vi "CloseBuild.vi"(8 "error in (no error)":errorcluster, 9 "GeneratedFiles":path[](array[path]), 10 "GeneratedDirectories":path[](array[path]), 11 "Build in":refnum<class "AB_Targetfile.lvclass">) -> (0 "error out":errorcluster, 1 "GeneratedFiles out":path[](array[path]), 3 "Build out":refnum<class "AB_Targetfile.lvclass">)   [LabVIEW 2020, in "AB_Targetfile.lvclass"]
uses:
  <vilib>/AppBuilder/AB_Classes/TargetFile/AB_Targetfile.lvclass
  e:/builds/penguin/labview/branches/2020/dev/dist/vi.lib/AppBuilder/AB_Classes/Build/AB_Build.lvclass
  <vilib>/Utility/error.llb/whitespace.ctl
  <vilib>/AppBuilder/AB_Classes/Build/AB_Build.lvclass
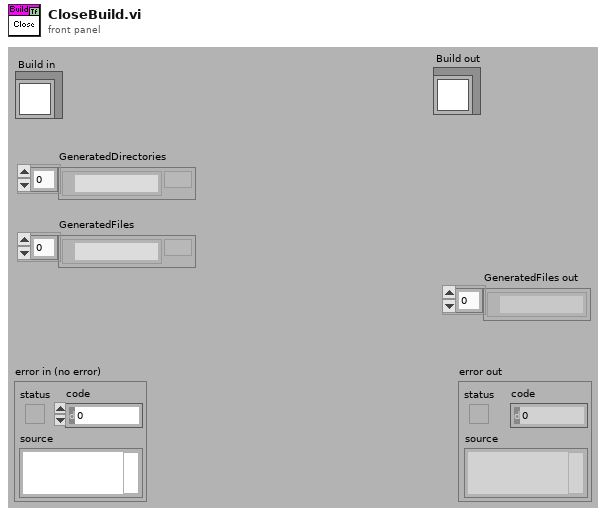
[diagram p1: front panel]
types:
  T1 = typedef "AB_Build.ctl" = cluster{"buildSpecName":string, "buildSpecDescription":string, "destinations":refnum<class "AB_Destination.lvclass">[], "exclusionOption":T2, "defaultLanguage":string, "supportedLanguages":string[], "excludedDirectories":path[], "buildContext":refnum<vi>, "buildObject":T3, "preview":bool, "programatic":bool, "progressBarEvents":T4, "userLog_Path":path, "preActionID":string, "preAction_Path":path, "postActionID":string, "postAction_Path":path, "eng_checkForBrokenVIs?":bool, "eng_verboseLinkerErrors?":bool, "localDest_Path":path, "targetDest_Path":path, "removeVIObject":u16, "cache":refnum<class "PreviewCache.lvclass">, "use cache":bool, "previewCache_ID":string, "buildCache_ID":string, "eng_TempLocalDest_Path":path, "eng_collectDependencies?":bool, "versionInfo":cluster{"buildVersion":cluster{"major":u16, "minor":u16, "patch":u16, "build":u16}, "autoIncrement":bool}, "eng_enableVIChecksums":bool}
  T2 = typedef "AB_Exclusion_Option.ctl" = cluster{"typedefs":bool, "polymorphicVIs":bool, "unusedLibraryItems":bool, "modifyLibraryFile":bool, "edit-timeDependencies":bool, "inlineVIs":bool, "dependent PPLs":bool, "dependent DLLs":bool}
  T3 = typedef "ItemRef.ctl" = u64
  T4 = typedef "provcom_ProgressBar_Events.ctl" = cluster{"newJob":refnum<user-event>, "newItem":refnum<user-event>, "errorMsg":T5, "cancel":refnum<user-event>}
  T5 = typedef "mxLvBuildError.ctl" = refnum<user-event>
  T6 = cluster{"major":u16, "minor":u16, "patch":u16, "build":u16}
  T7 = typedef "AB_Targetfile.ctl" = cluster{"targetfileName":string, "targetfileGUID":string, "enableDebugging":bool, "versionInfo":cluster{"productName":string, "legalCopyright":string, "companyName":string, "internalName":string, "fileDescription":string}, "eng_consolidatedTypeInfo":string, "fastFileFormat":bool, "eng_LEIFBuildData":u32, "versionIndependent":bool}
  T8 = typedef "whitespace.ctl" = u16
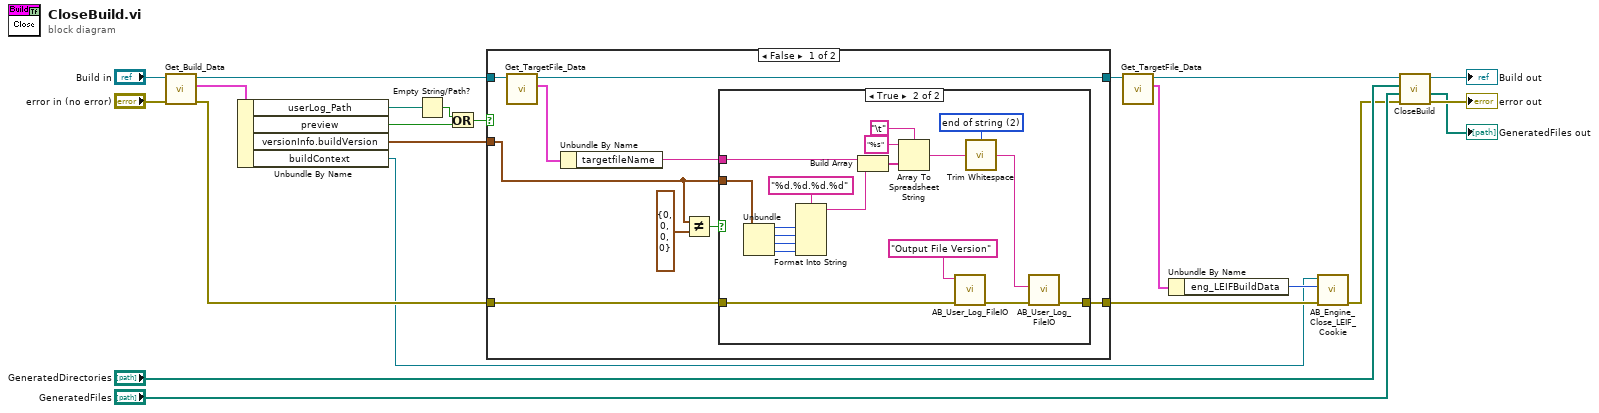
[diagram p0: block diagram]
diagram:
  n1 = call <vilib>:"Get_Build_Data.vi"("error in (no error)"="error in (no error)", "Class in"="Build in") -> ("error out"=w13:errorcluster, "data"=w14:T1, "Class out"=w12:refnum<class "AB_Targetfile.lvclass">)  [unwired: 7 out]
  n2 = Unbundle By Name(w14) -> ("userLog_Path"=w17:path, "preview"=w11:bool, "versionInfo.buildVersion"=w8:T6, "buildContext"=w1:refnum<vi>)
  n3 = Empty String/Path?(string/path=w17) -> (empty?=w10:bool)
  n4 = Or(x=w10, y=w11) -> (x .or. y?=w9:bool)
  n5 = case shown="False" w9 {
    tunnel: w13 -> [w30 w52]
    tunnel: [w31 w52] -> w4
    tunnel: w12 -> [w29 w51]
    tunnel: [w28 w51] -> w7
    tunnel: w8 -> [w23 _]
    frame False {
      n6 = call <vilib>:"Get_TargetFile_Data.vi"("AB_Targetfile in"=w29) -> ("data"=w27:T7, "AB_Targetfile out"=w28:refnum<class "AB_Targetfile.lvclass">)  [unwired: 8 in, 1 out]
      n7 = Unbundle By Name(w27) -> ("targetfileName"=w26:string)
      n8 = Not Equal?(x=w23, y=T6 {"major"=0, "minor"=0, "patch"=0, "build"=0} ("versionInfo.fileVersion")) -> (x != y?=w24:bool)
      n9 = case shown="True" w24 {
        tunnel: [w32 w50] -> w31
        tunnel: w30 -> [w32 w48]
        tunnel: w26 -> [_ w34]
        tunnel: w23 -> [_ w33]
        frame False {
          # "If the version info is default, don't write anything out. This is to guard web services from writing out a version since lvws files don't have them. While it may be possible to set the version of apps to all zeros, it isn't a very useful value."
        }
        frame True {
          w36 = T8 2 items=["both", "start of string", "end of string"] ("location (both)")
          n10 = Unbundle(w33) -> ("major"=w42:u16, "minor"=w41:u16, "patch"=w40:u16, "build"=w39:u16)
          n11 = Format Into String(format string="%d.%d.%d.%d", w42, w41, w40, w39) -> (resulting string=w38:string)  [unwired: 2 in, 1 out]
          n12 = Build Array(w34, w38) -> (w46:string[])
          n13 = Array To Spreadsheet String(delimiter (Tab)="\t", array=w46, 3:"%s" ("format string")) -> (spreadsheet string=w44:string)
          n14 = call <vilib>:"AB_User_Log_FileIO.vi"("error in (no error)"=w48, "newSection"="Output File Version") -> ("error out"=w47:errorcluster)  [unwired: 3 in, 6 out]
          n15 = call <vilib>:"Trim Whitespace.vi"("string"=w44, "location (both)"=w36) -> ("trimmed string"=w37:string)
          n16 = call <vilib>:"AB_User_Log_FileIO.vi"("error in (no error)"=w47, "data"=w37) -> ("error out"=w50:errorcluster)  [unwired: 3 in, 6 out]
        }
      }
    }
    frame True {
    }
  }
  n17 = call <vilib>:"Get_TargetFile_Data.vi"("AB_Targetfile in"=w7) -> ("data"=w5:T7, "AB_Targetfile out"=w6:refnum<class "AB_Targetfile.lvclass">)  [unwired: 8 in, 1 out]
  n18 = Unbundle By Name(w5) -> ("eng_LEIFBuildData"=w2:u32)
  n19 = call <vilib>:"AB_Engine_Close_LEIF_Cookie.vi"("error in (no error)"=w4, "eng_LEIFBuildData"=w2, "buildContext"=w1) -> ("error out"=w3:errorcluster)  [unwired: 8 in]
  n20 = call-parent "CloseBuild.vi"("error in (no error)"=w3, "GeneratedFiles"="GeneratedFiles", "GeneratedDirectories"="GeneratedDirectories", "Build in"=w6) -> ("error out"=→"error out":errorcluster, "GeneratedFiles out"=→"GeneratedFiles out":path[], "Build out"=→"Build out":refnum<class "AB_Targetfile.lvclass">)  [unwired: 5 out]
